vi "Read Jitter Measurement (Data TIE).vi"(8 "error in (no error)":errorcluster, 9 "Units Data TIE (0: Seconds)":u16(ring) items=["Seconds", "Unit Interval"], 10 "Source Data TIE (0: Channel 1)":u16(ring) items=["Channel 1", "Channel 2", "Channel 3", "Channel 4", "Math 1", "Math 2", "Math 3", "Math 4", "Reference Waveform 1", "Reference Waveform 2", "Reference Waveform 3", "Reference Waveform 4"], 11 "VISA resource name":refnum<visa-resource-name>) -> (0 "error out":errorcluster, 2 "Data TIE":dbl, 3 "VISA resource name out":refnum<visa-resource-name>)   [LabVIEW 2017, in "Agilent 2000 3000 X-Series.lvlib"]
doc: "Measures and returns the Data TIE jitter value.\n\n<b>Note:</b>\nThis VI is specific to the 6000-X Series oscilloscopes. These features are not available on other models."
uses:
  Agilent 2000 3000 X-Series.lvlib
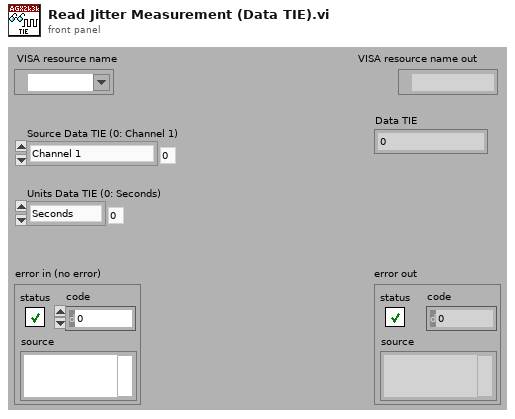
[diagram p1: front panel]
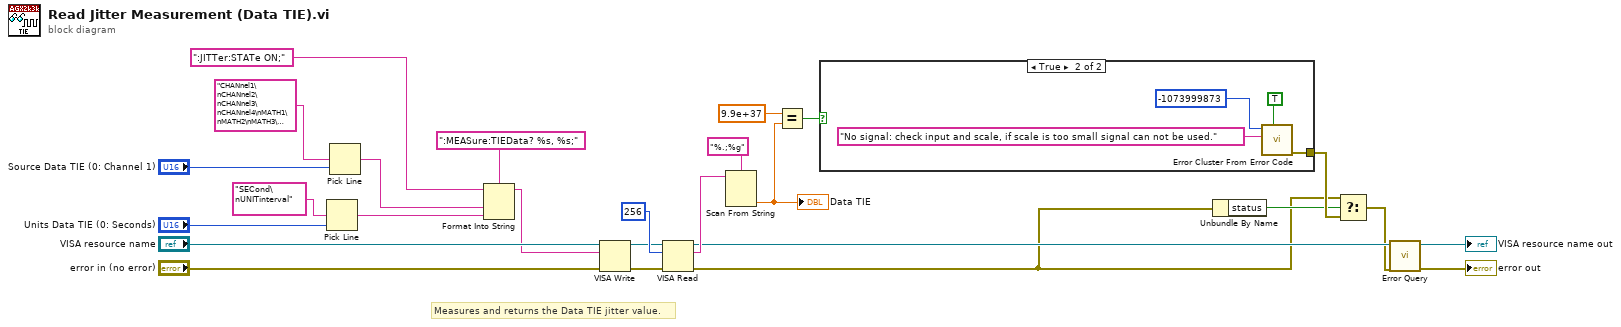
[diagram p0: block diagram]
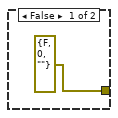
[diagram p2: hidden frame]
diagram:
  # "Measures and returns the Data TIE jitter value."
  n1 = Pick Line(multi-line string="SECond\nUNITinterval", line index="Units Data TIE (0: Seconds)") -> (output string=w23:string)  [unwired: 1 in]
  n2 = Pick Line(multi-line string="CHANnel1\nCHANnel2\nCHANnel3\nCHANnel4\nMATH1\nMATH2\nMATH3\nMATH4\nWMEMory1\nWMEMory2\nWMEMory3\nWMEMory4", line index="Source Data TIE (0: Channel 1)") -> (output string=w26:string)  [unwired: 1 in]
  n3 = Format Into String(format string=":MEASure:TIEData? %s, %s;", initial string=":JITTer:STATe ON;", w26, w23) -> (resulting string=w15:string)  [unwired: 1 in, 1 out]
  n4 = VISA Write(VISA resource name="VISA resource name", write buffer=w15, error in (no error)="error in (no error)") -> (VISA resource name out=w9:refnum<visa-resource-name>, error out=w10:errorcluster)  [unwired: 1 out]
  n5 = VISA Read(VISA resource name=w9, byte count=u32 256, error in (no error)=w10) -> (VISA resource name out=w11:refnum<visa-resource-name>, read buffer=w12:string, error out=w2:errorcluster)  [unwired: 1 out]
  n6 = Scan From String(format string="%.;%g", input string=w12) -> (output 1=w5:dbl)  [unwired: 3 in, 3 out]
  "Data TIE" <- w5
  n7 = Equal?(x=9.9e+37, y=w5) -> (x = y?=w8:bool)
  n8 = case shown="True" w8 {
    tunnel: [errorcluster {"status"=FALSE, "code"=0, "source"=""} ("error out") w28] -> w6
    frame False {
    }
    frame True {
      n9 = call <vilib>:"Error Cluster From Error Code.vi"("show call chain? (False)"=TRUE, "error message (\"\")"="No signal: check input and scale, if scale is too small signal can not be used." ("error message (\"\")"), "error code (0)"=-1073999873) -> ("error out"=w28:errorcluster)  [unwired: 6 in]
    }
  }
  n10 = Unbundle By Name(w2) -> ("status"=w4:bool)
  n11 = Select(t=w2, s=w4, f=w6) -> (s? t:f=w3:errorcluster)
  n12 = call "Error Query.vi"("error in (no error)"=w3, "VISA resource name"=w11) -> ("error out"=→"error out":errorcluster, "VISA resource name out"=→"VISA resource name out":refnum<visa-resource-name>)  [unwired: 6 in, 2 out]
